vi "Date_and_Time_to_string.vi"() -> (0 "Date and time (spreadsheet)":string)   [LabVIEW 2015]
uses:
  Globals/Preference_global.vi
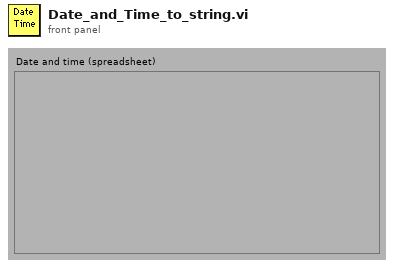
[diagram p1: front panel]
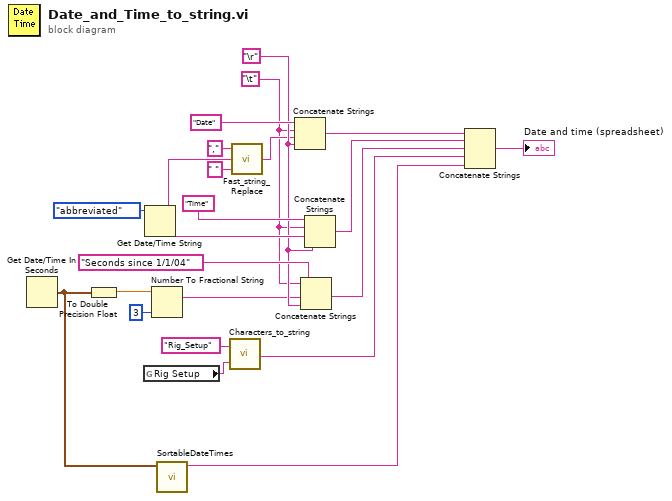
[diagram p0: block diagram]
diagram:
  w12 = "\r"
  w2 = "\t"
  n1 = Get Date/Time In Seconds() -> (seconds since 1Jan1904=w3:timestamp)
  n2 = To Double Precision Float(number=w3) -> (double precision float=w10:dbl)
  n3 = global read "Preference_global.vi" "Rig Setup"() -> (w11:string)
  n4 = Get Date/Time String(date format (0)=enum16{"short", "long", "abbreviated"}."abbreviated") -> (date string=w7:string, time string=w21:string)  [unwired: 2 out]
  n5 = Number To Fractional String(number=w10, precision (6)=i16 3) -> (F-format string=w8:string)  [unwired: 2 out]
  n6 = call "SortableDateTimes.vi"("seconds since 1Jan1904"=w3) -> ("SortableDate-Times"=w1:string)  [unwired: 10 in]
  n7 = call "Characters_to_string.vi"("Characters to write"=w11, "Label for characters"="Rig_Setup") -> ("Output string"=w13:string)
  n8 = call "Fast_string_Replace.vi"("Replace match with:"=" ", "Input String"=w7, "regular expression"=",") -> ("Output String"=w6:string)  [unwired: 2 out]
  n9 = Concatenate Strings("Date", w2, w6, w12) -> (w20:string)
  n10 = Concatenate Strings("Seconds since 1/1/04", w2, w8, w12) -> (w17:string)
  n11 = Concatenate Strings("Time", w2, w21, w12) -> (w19:string)
  n12 = Concatenate Strings(w20, w19, w17, w13, w1) -> (→"Date and time (spreadsheet)":string)
